vi "Host-OrderBook-SendData.vi"(8 "error in":errorcluster, 10 "FPGA VI Reference in":T1, 11 "OrderBook-Commands":T2(array[cluster]) {"Cluster"."OrderRefNum" format="%.0x"}) -> (0 "error out":errorcluster, 3 "FPGA VI Reference out":T1)   [LabVIEW 2016]
uses:
  OrderBook-TestHarness-Typedef.ctl
  <vilib>/rvi/interface/RandomDataEmulation/nirviRandomDataDMAMethods.vi
  <vilib>/rvi/interface/nirviMethod/nirviMethod.xnode
  Fpga/Tests/Fpga-OrderBook-TestHarness.vi
panel:
  out "Array":u8[][](array[numeric])
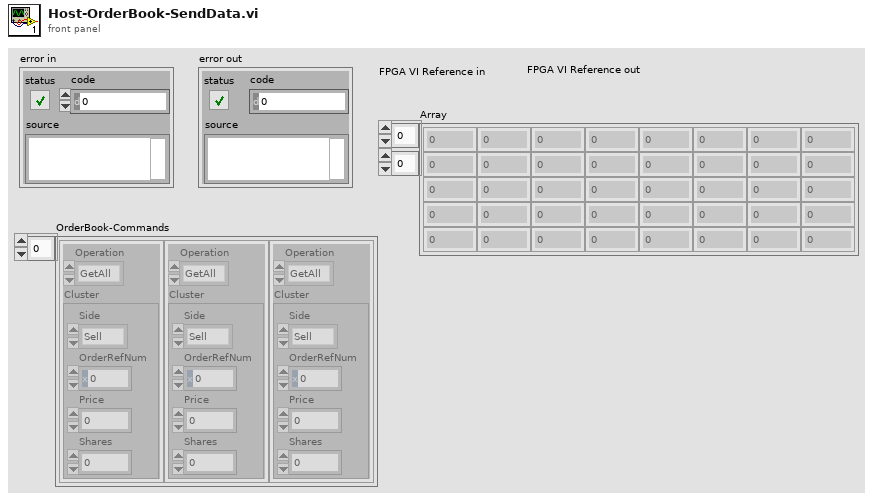
[diagram p1: front panel]
types:
  T1 = typedef "OrderBook-TestHarness-Typedef.ctl" = refnum<k20>
  T2 = cluster{"Operation":enum16{"Noop", "GetAll", "AddOrder", "DeleteOrder"}, "Cluster":cluster{"Side":enum16{"Sell", "Buy"}, "OrderRefNum":u64, "Price":u32, "Shares":u32}}[]
  T3 = enum16{"Noop", "GetAll", "AddOrder", "DeleteOrder"}
  T4 = cluster{"Side":enum16{"Sell", "Buy"}, "OrderRefNum":u64, "Price":u32, "Shares":u32}
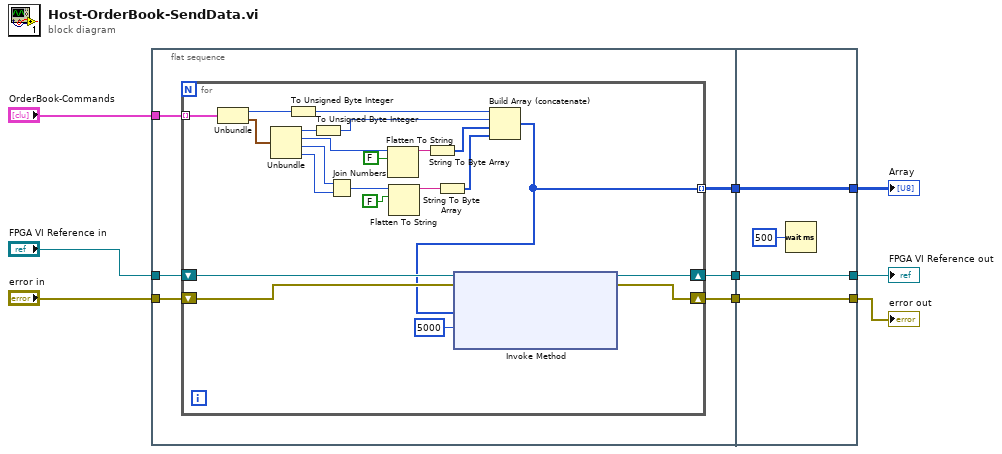
[diagram p0: block diagram]
diagram:
  n1 = flat-sequence {
    tunnel: "OrderBook-Commands" -> [w15]
    tunnel: "error in" -> [w13]
    tunnel: "FPGA VI Reference in" -> [w12]
    tunnel: [w14] -> w3
    tunnel: [w11] -> w2
    tunnel: [w10] -> w1
    tunnel: [w39] -> w4
    tunnel: [w40] -> w5
    tunnel: [w41] -> w8
    tunnel: w3 -> [w41]
    tunnel: w2 -> [w40]
    tunnel: w1 -> [w39]
    frame #0 {
      n2 = for {
        tunnel: w15 -> [w37] mode=indexing
        shift-right: [w36] -> w11
        shift-left: w12 -> [w33]
        shift-right: [w35] -> w14
        shift-left: w13 -> [w34]
        tunnel: [w16] -> w10 mode=indexing
        n3 = Unbundle(w37) -> ("Operation"=w32:T3, "Cluster"=w30:T4)
        n4 = Unbundle(w30) -> ("Side"=w29:enum16{"Sell", "Buy"}, "OrderRefNum"=w27:u64, "Price"=w23:u32, "Shares"=w22:u32)
        n5 = To Unsigned Byte Integer(number=w32) -> (unsigned 8bit integer=w31:u8)
        n6 = To Unsigned Byte Integer(number=w29) -> (unsigned 8bit integer=w28:u8)
        n7 = Join Numbers(hi=w23, lo=w22) -> ((hi.lo)=w20:u64)
        n8 = Flatten To String(anything=w27, prepend array or string size? (T)=FALSE) -> (data string=w25:string)  [unwired: 2 in, 2 out]
        n9 = Flatten To String(anything=w20, prepend array or string size? (T)=FALSE) -> (data string=w19:string)  [unwired: 2 in, 2 out]
        n10 = String To Byte Array(string=w25) -> (unsigned byte array=w24:u8[])
        n11 = String To Byte Array(string=w19) -> (unsigned byte array=w18:u8[])
        n12 = Build Array (concatenate)(w31, w28, w24, w18) -> (w16:u8[])
        n13 = xnode "Invoke Method"("FPGA VI Reference In"=w33, "error in"=w34, "Data"=w16, "Timeout (ms)"=5000) -> ("FPGA VI Reference Out"=w36:T1, "error out"=w35:errorcluster)  [unwired: 1 out]
      }
    }
    frame #1 {
      n14 = Wait (ms)(milliseconds to wait=u32 500) -> ()  [unwired: 1 out]
    }
  }
  "error out" <- w8
  "FPGA VI Reference out" <- w5
  "Array" <- w4
